vi "Increment Date.vi"(8 "error in (no error)":errorcluster, 11 "Budgetizer in":refnum<class "Budgetizer.lvclass">) -> (0 "error out":errorcluster, 3 "Budgetizer out":refnum<class "Budgetizer.lvclass">)   [LabVIEW 2018, in "Budgetizer.lvclass"]
uses:
  Budgetizer.lvclass
  Budgetizer.lvclass/Budgetizer.ctl
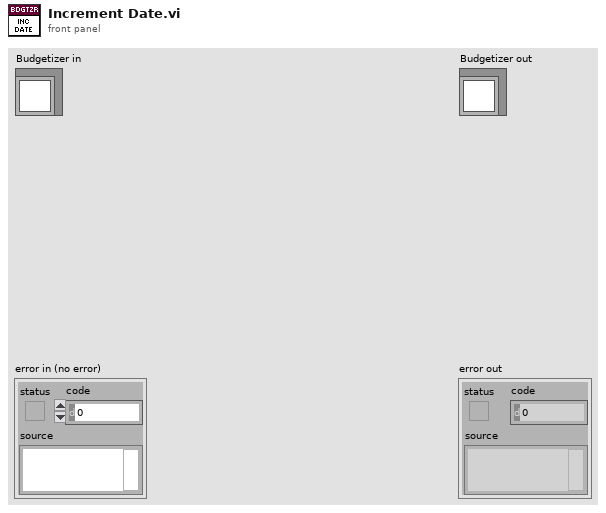
[diagram p1: front panel]
types:
  T1 = enum16{"January", "February", "March", "April", "May", "June", "July", "August", "September", "October", "November", "December"}
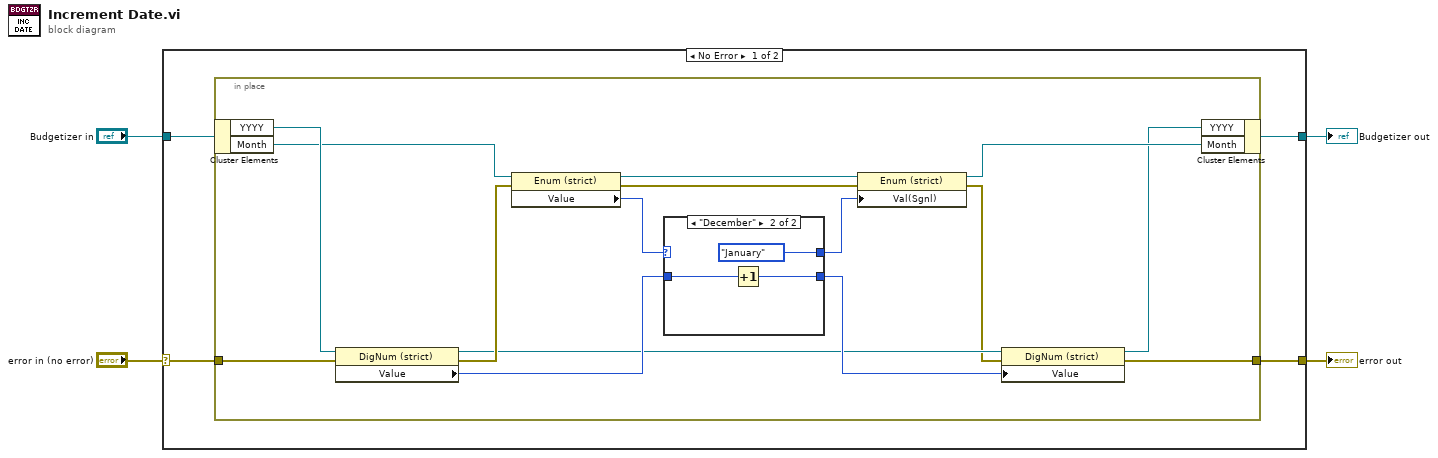
[diagram p0: block diagram]
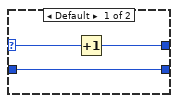
[diagram p2: hidden frame]
diagram:
  n1 = case shown="No Error" "error in (no error)" {
    selector: "error in (no error)" -> [w7 w31]
    tunnel: [w5 w31] -> w3
    tunnel: [w6 w30] -> w1
    tunnel: "Budgetizer in" -> [w8 w30]
    frame No Error {
      n2 = in-place {
        in-place-border: w7 -> [w19]
        in-place-border: [w9] -> w5
        n3 = in-place-cluster #1(w8) -> ("YYYY"=w20:refnum<vi>, "Month"=w18:refnum<vi>)
        n4 = property on="Property Node" class="DigNum (strict)"(reference=w20, error in=w19) -> (reference out=w12:refnum<vi>, error out=w21:errorcluster, "Value"=w16:i32)
        n5 = property on="Property Node" class="Enum (strict)"(reference=w18, error in=w21) -> (reference out=w14:refnum<vi>, error out=w15:errorcluster, "Value"=w17:T1)
        n6 = case shown="\"December\"" w17 {
          selector: w17 -> [w26 _]
          tunnel: w16 -> [w25 w28]
          tunnel: [w25 w27] -> w23
          tunnel: [w24 T1."January"] -> w22
          frame Default {
            n7 = Increment(x=w26) -> (x+1=w24:T1)
          }
          frame "December" {
            n8 = Increment(x=w28) -> (x+1=w27:i32)
          }
        }
        n9 = property on="Property Node" class="Enum (strict)"(reference=w14, error in=w15, "Val(Sgnl)"=w22) -> (reference out=w13:refnum<vi>, error out=w11:errorcluster)
        n10 = property on="Property Node" class="DigNum (strict)"(reference=w12, error in=w11, "Value"=w23) -> (reference out=w10:refnum<vi>, error out=w9:errorcluster)
        n11 = in-place-cluster #1("YYYY"=w10, "Month"=w13) -> (w6:refnum<class "Budgetizer.lvclass">)
      }
    }
    frame Error {
    }
  }
  "error out" <- w3
  "Budgetizer out" <- w1
